vi "I-AC-global.vi"() -> ()   [LabVIEW 2013]
panel:
  in  "AC Current Array":dbl[](array[numeric])
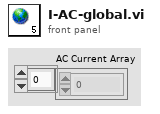
[diagram p1: front panel]
diagram:
